vi "GrahamRobertsW01052583Lab7.vi"() -> ()   [LabVIEW 2014]
panel:
  in  "stop":bool
  in  "run":bool
  out "average":dbl
  out "trials":dbl
  out "total":dbl
  in  "measurement":dbl
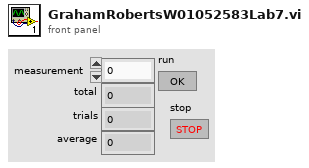
[diagram p1: front panel]
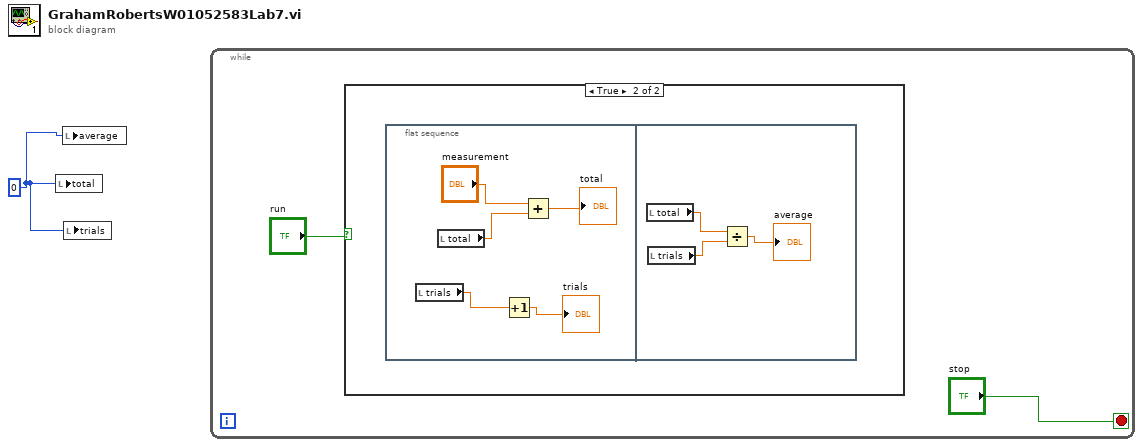
[diagram p0: block diagram]
diagram:
  w1 = 0
  n1 = local write "total"(w1) -> ()
  n2 = local write "average"(w1) -> ()
  n3 = local write "trials"(w1) -> ()
  n4 = while {
    stop <- "stop" stop-if-true
    n5 = case shown="True" "run" {
      frame False {
      }
      frame True {
        n6 = flat-sequence {
          frame #0 {
            n7 = local read "trials"() -> (w6:dbl)
            n8 = local read "total"() -> (w4:dbl)
            n9 = Increment(x=w6) -> (x+1=→"trials":dbl)
            n10 = Add(x="measurement", y=w4) -> (x+y=→"total":dbl)
          }
          frame #1 {
            n11 = local read "total"() -> (w11:dbl)
            n12 = local read "trials"() -> (w10:dbl)
            n13 = Divide(x=w11, y=w10) -> (x/y=→"average":dbl)
          }
        }
      }
    }
  }
